vi "DisplayLogic_DrawAstronaut.vi"(2 "ActivePixel":cluster{"h_pixel":i16, "v_pixel":i16}) -> (16 "PixelData":bool[](array[boolean]))   [LabVIEW 2018]
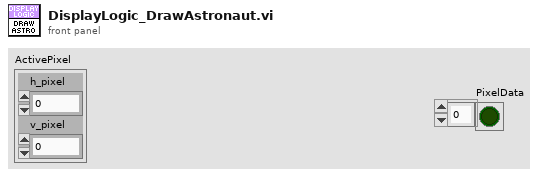
[diagram p1: front panel]
types:
  T1 = cluster{"left":i16, "top":i16, "right":i16, "bottom":i16}
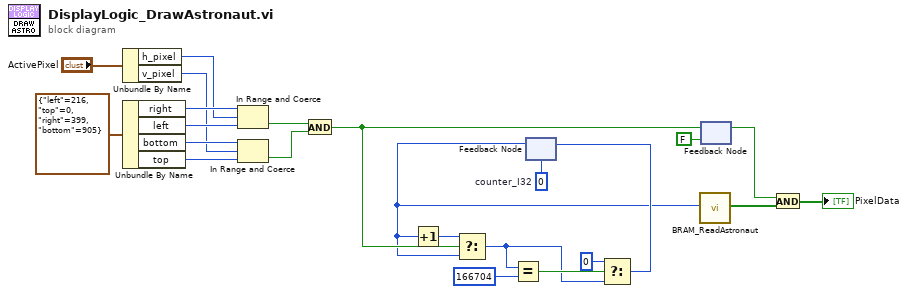
[diagram p0: block diagram]
diagram:
  w14 = 0  # counter_I32
  n1 = Unbundle By Name("ActivePixel") -> ("h_pixel"=w5:i16, "v_pixel"=w4:i16)
  n2 = Unbundle By Name(T1 {"left"=216, "top"=0, "right"=399, "bottom"=905}) -> ("right"=w19:i16, "left"=w23:i16, "bottom"=w17:i16, "top"=w20:i16)
  n3 = In Range and Coerce(upper limit=w19, x=w5, lower limit=w23) -> (In Range?=w22:bool)  [unwired: 1 out]
  n4 = In Range and Coerce(upper limit=w17, x=w4, lower limit=w20) -> (In Range?=w21:bool)  [unwired: 1 out]
  n5 = And(x=w22, y=w21) -> (x .and. y?=w10:bool)
  n6 = feedback #1(w14) -> (w7:i32)
  n7 = Increment(x=w7) -> (x+1=w12:i32)
  n8 = Select(t=w12, s=w10, f=w7) -> (s? t:f=w11:i32)
  n9 = Equal?(x=w11, y=166704) -> (x = y?=w13:bool)
  n10 = Select(t=0 ("f"), s=w13, f=w11) -> (s? t:f=w16:i32)
  n11 = feedback-in #1(w16) -> ()
  n12 = call "BRAM_ReadAstronaut.vi"("Address"=w7) -> ("PixelData"=w3:bool[])  [unwired: 18 in]
  n13 = feedback #2(FALSE) -> (w2:bool)
  n14 = feedback-in #2(w10) -> ()
  n15 = And(x=w2, y=w3) -> (x .and. y?=→"PixelData":bool[])
